vi "TEST_ALL.vi"() -> ()   [LabVIEW 2013]
uses:
  Test State.ctl
  ValveDefaults.ctl
  <vilib>/DAQmx/read.llb/DAQmx Read (Counter DBL 1Chan 1Samp).vi
  <vilib>/DAQmx/read.llb/DAQmx Read (Analog 1D Wfm NChan NSamp).vi
  <vilib>/DAQmx/configure/timing.llb/DAQmx Timing (Sample Clock).vi
  <vilib>/DAQmx/miscellaneous.llb/DAQmx Fill In Error Info.vi
panel:
  in  "Fuel Type":enum16{"RP1", "Biodiesel", "Water"}(ring)=enum."Biodiesel"
  in  "Oxidizer Type":enum16{"LOX", "Water", "Nitrogen"}(ring)
  out "Specific Impulse Display":waveform(dbl)(graph)={"t0"=timestamp(3577994788.047329 s since 1904-01-01), "dt"=0.001, "Y"=[0.0, 0.0, 0.0, 0.0, 0.0, 0.0, 0.0, 0.0, 0.0, 0.0, 0.0, 0.0, 0.0, 0.0, 0.0, 0.0, 0.0, 0.0, 0.0, 0.0, 0.0, 0.0, 0.0, 0.0, 0.0, 0.0, 0.0, 0.0, 0.0, 0.0, 0.0, 0.0, 0.0, 0.0, 0.0, 0.0, 0.0, 0.0, 0.0, 0.0, 0.0, 0.0, 0.0, 0.0, 0.0, 0.0, 0.0, 0.0, 0.0, 0.0, 0.0, 0.0, 0.0, 0.0, 0.0, 0.0, 0.0, 0.0, 0.0, 0.0, 0.0, 0.0, 0.0, 0.0, 0.0, 0.0, 0.0, 0.0, 0.0, 0.0, 0.0, 0.0, 0.0, 0.0, 0.0, 0.0, 0.0, 0.0, 0.0, 0.0, 0.0, 0.0, 0.0, 0.0, 0.0, 0.0, 0.0, 0.0, 0.0, 0.0, 0.0, 0.0, 0.0, 0.0, 0.0, 0.0, 0.0, 0.0, 0.0, 0.0], "attributes"=variant("NI_ChannelName"=variant(string "Loadcell5k"), "NI_UnitDescription"=variant(string "lbs"))} caption="Measurement"
  in  "Burn Time":dbl=6.0
  out "LOX Rate":dbl
  out "Fuel Rate":dbl
  in  "Loop Freq (Hz)":i32=10
  out "LOX Flow Count":dbl
  out "Fuel Flow Count":dbl
  in  "Maximum Pressures":dbl[](array[numeric])=[600.0, 600.0, 600.0, 600.0, 600.0]
  out "Engine Pressure":waveform(dbl)(graph)={"t0"=timestamp(3577994788.047329 s since 1904-01-01), "dt"=0.001, "Y"=[0.0, 0.0, 0.0, 0.0, 0.0, 0.0, 0.0, 0.0, 0.0, 0.0, 0.0, 0.0, 0.0, 0.0, 0.0, 0.0, 0.0, 0.0, 0.0, 0.0, 0.0, 0.0, 0.0, 0.0, 0.0, 0.0, 0.0, 0.0, 0.0, 0.0, 0.0, 0.0, 0.0, 0.0, 0.0, 0.0, 0.0, 0.0, 0.0, 0.0, 0.0, 0.0, 0.0, 0.0, 0.0, 0.0, 0.0, 0.0, 0.0, 0.0, 0.0, 0.0, 0.0, 0.0, 0.0, 0.0, 0.0, 0.0, 0.0, 0.0, 0.0, 0.0, 0.0, 0.0, 0.0, 0.0, 0.0, 0.0, 0.0, 0.0, 0.0, 0.0, 0.0, 0.0, 0.0, 0.0, 0.0, 0.0, 0.0, 0.0, 0.0, 0.0, 0.0, 0.0, 0.0, 0.0, 0.0, 0.0, 0.0, 0.0, 0.0, 0.0, 0.0, 0.0, 0.0, 0.0, 0.0, 0.0, 0.0, 0.0], "attributes"=variant("NI_ChannelName"=variant(string "Loadcell5k"), "NI_UnitDescription"=variant(string "lbs"))} caption="Measurement"
  in  "Write Data Button":bool
  out "Test Message":string
  in  "Start Test Button":bool
  in  "Abort Button":bool
  out "Armed Light":bool
  in  "Fire Button":bool
  in  "ARM TEST":bool
  out "Test State":T1
  out "Load Cell Display":waveform(dbl)(graph) caption="Measurement"
  out "Thermocouple 2 Num":dbl
  out "Thermocouple 1 Num":dbl
  in  "Max Temp 2":dbl=500.0
  in  "Max Temp 1":dbl=500.0
  out "LOX Temp":dbl(slide) scale=-200.0..-100.0
  out "Fuel Temp":dbl(slide) scale=-50.0..50.0
  out "Caution 3":bool
  out "Overtemp Alert":bool
  out "Caution 2":bool
  out "Saving Data Alert":bool
  out "Overpressure Alert":bool
  in  "Analog Data Filepath":path=path "C:/MAE155B-Data/analog-test-data.lvm"
  in  "Sample Rate":dbl=1000.0 caption="Analog Rate (Hz)" format="%0.2f"
  in  "Samples to Read":i32=100 caption="Analog Samples"
  out "LOX Dome Pressure":dbl(knob) scale=0.0..600.0
  out "Fuel Dome Pressure":dbl(knob) scale=0.0..600.0
  out "LOX Tank Pressure":dbl(knob) scale=0.0..600.0
  out "Fuel Tank Pressure":dbl(knob) scale=0.0..600.0
  out "AIR BLEED STATUS":bool
  in  "STOP ALL BUTTON 2":bool
  out "LOX VALVE STATUS":bool
  out "LOX DOME OUT STATUS":bool
  out "LOX DOME IN STATUS":bool
  out "VENT STATUS":bool
  out "FUEL VALVE STATUS":bool
  out "FUEL DOME OUT STATUS":bool
  out "FUEL DOME IN STATUS":bool
  in  "LOX DOME IN":bool
  in  "LOX DOME OUT":bool
  in  "AIR BLEED":bool=TRUE
  in  "FUEL DOME IN":bool
  in  "VENT":bool=TRUE
  in  "LOX VALVE":bool
  in  "FUEL DOME OUT":bool
  in  "FUEL VALVE":bool
  out "LOX Tank (gal)":dbl(slide) scale=0.0..3.0
  out "Fuel Tank (gal)":dbl(slide) scale=0.0..3.0
  # "VALVES WILL DEFAULT TO THEIR \"IDLE\" (NOT FAILURE) STATES WHEN PROGRAM STARTS.\nPRESS \"STOP ALL\" OR \"ABORT\" TO SEND VALVES TO THEIR FAILURE (NOT NECESSARILY UNPOWERED) STATES."
  # "DATA CONFIG"
  # "ANNUNCIATOR"
  # "All lights must be OFF before starting test!"
  # "TANK LEVELS"
  # "TEMPERATURES"
  # "VALVE CONTROL"
  # "TANK PRESSURE"
  # "EN"
  # "FT"
  # "FD"
  # "LT"
  # "LD"
  # "ENGINE PRESSURE"
  # "LOAD CELL"
  # "TEST STATE"
  # "MESSAGE"
  # "SPECIFIC IMPULSE"
  # "ARM TEST"
  # "TO DO: Fix the range on Isp graph!"
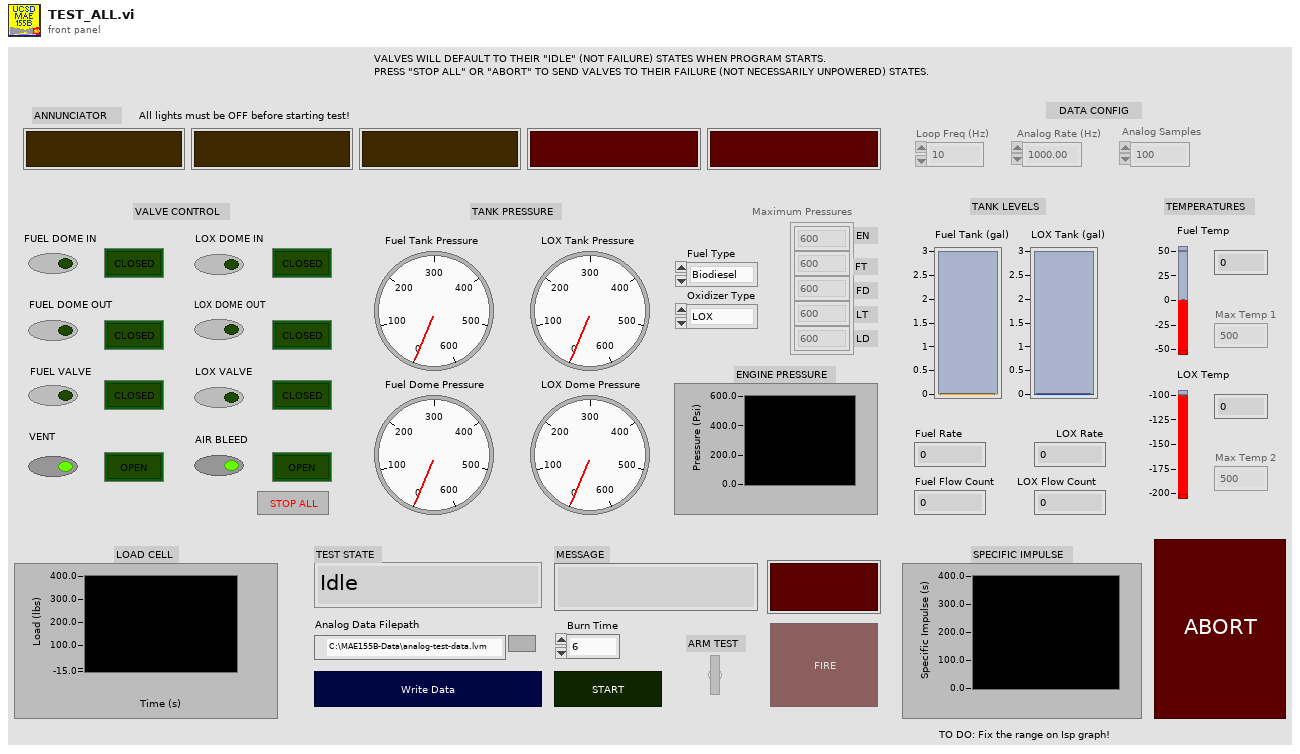
[diagram p1: front panel]
types:
  T1 = typedef "Test State.ctl" = enum16{"Idle", "Start", "LOX Valve Open", "Valve Open Wait", "Fuel Valve Open", "Burn Wait", "LOX Valve Close", "Valve Close Wait", "Fuel Valve Close", "Zero Dome", "Zero Wait", "Vent Valves Open", "Cooldown", "End"}
  T2 = typedef "ValveDefaults.ctl" = bool[]
  T3 = enum8{"Enabled", "Disabled", "Disabled and Grayed Out"}
  T4 = enum16{"NULL", "Caution Data", "Caution 2", "Caution 3", "Warning OverTemp", "Warning OverPressure"}
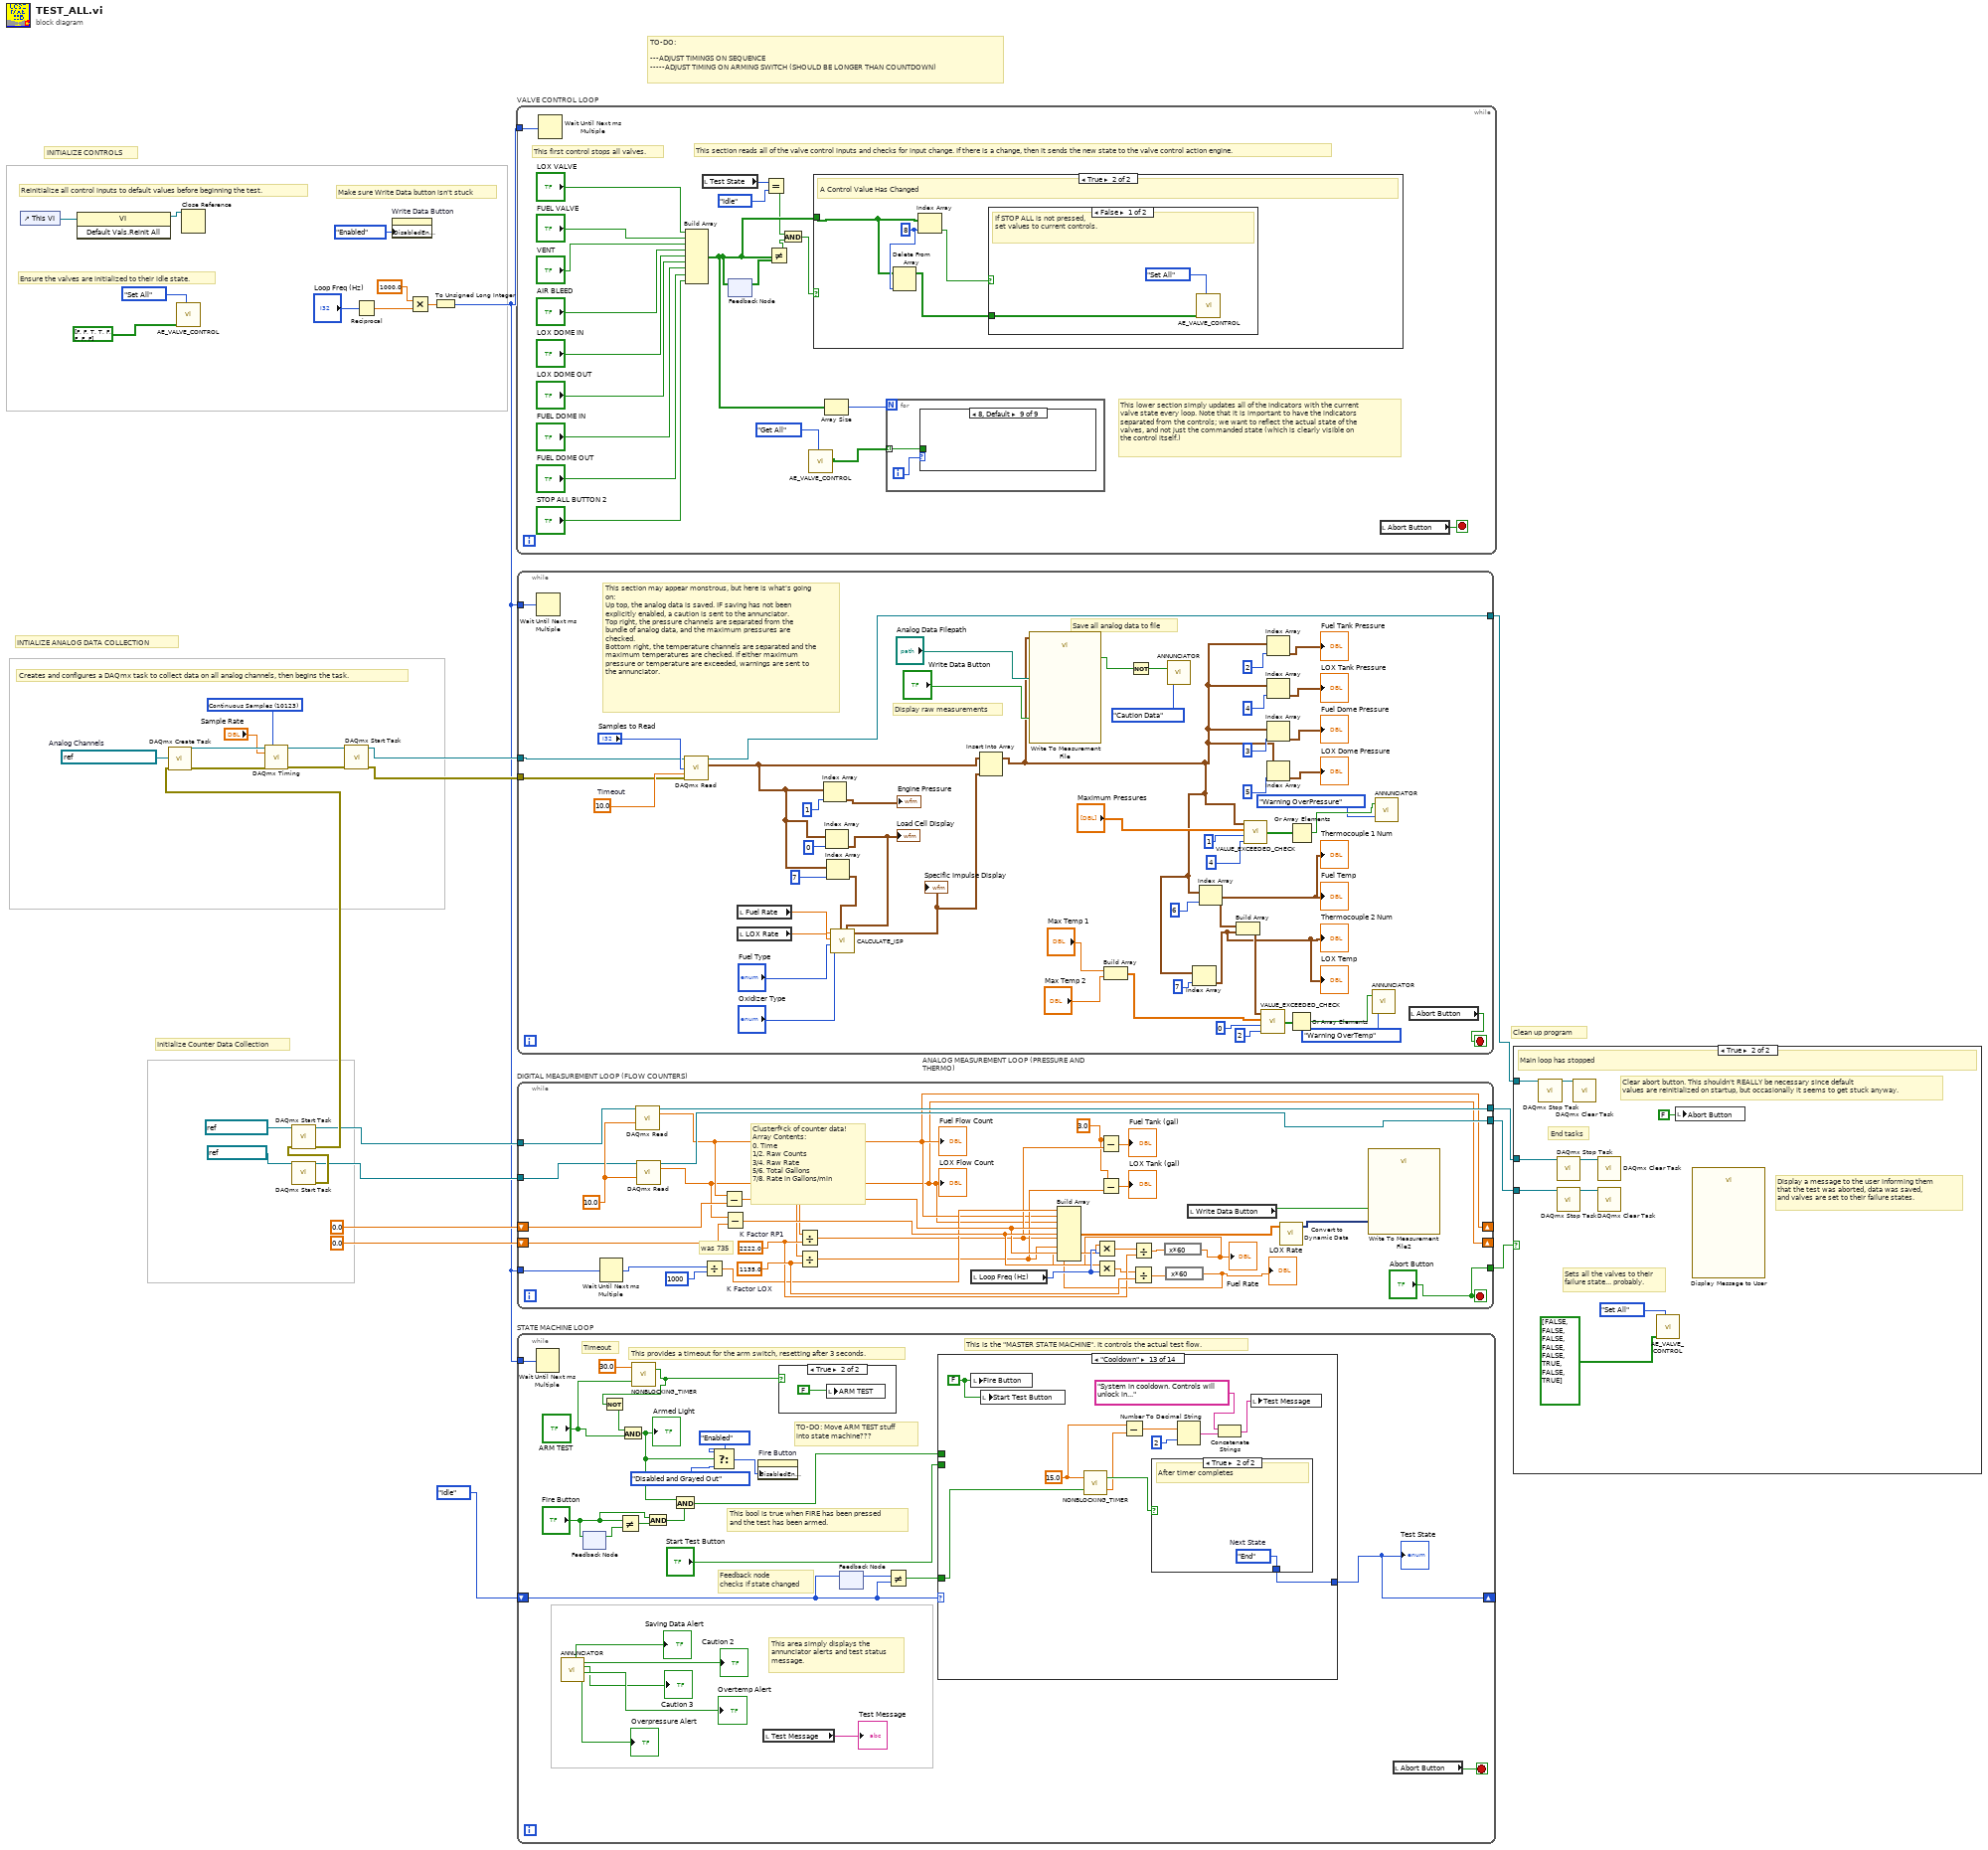
[diagram p0: block diagram]
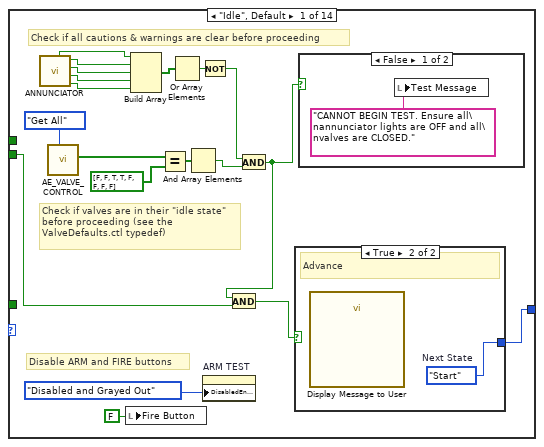
[diagram p2: hidden frame]
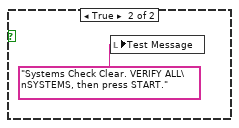
[diagram p3: hidden frame]
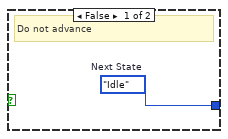
[diagram p4: hidden frame]
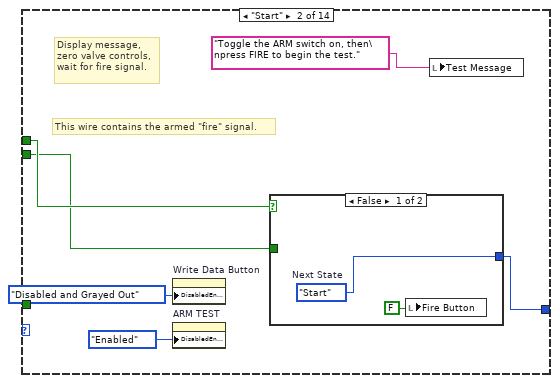
[diagram p5: hidden frame]
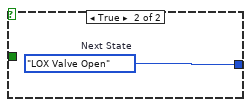
[diagram p6: hidden frame]
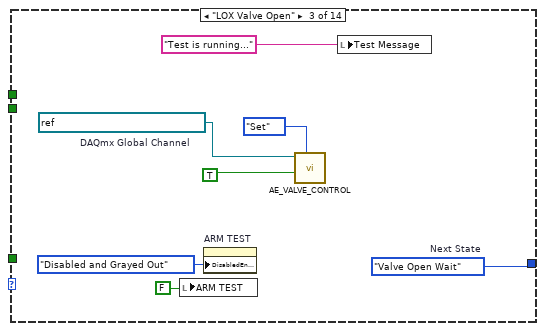
[diagram p7: hidden frame]
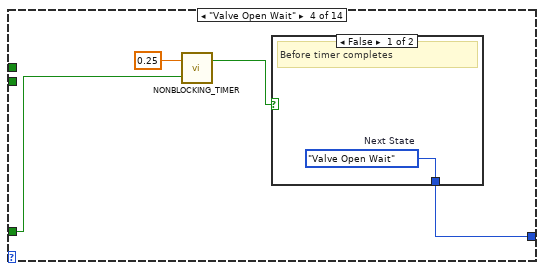
[diagram p8: hidden frame]
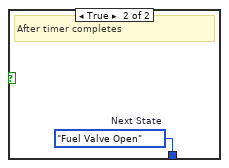
[diagram p9: hidden frame]
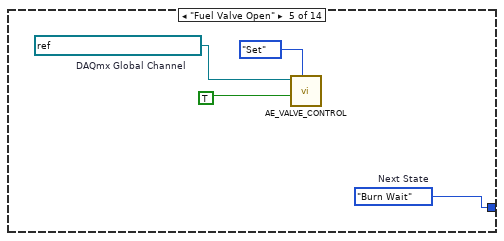
[diagram p10: hidden frame]
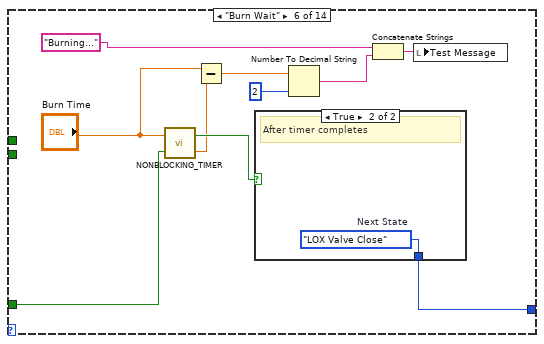
[diagram p11: hidden frame]
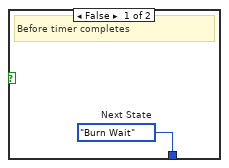
[diagram p12: hidden frame]
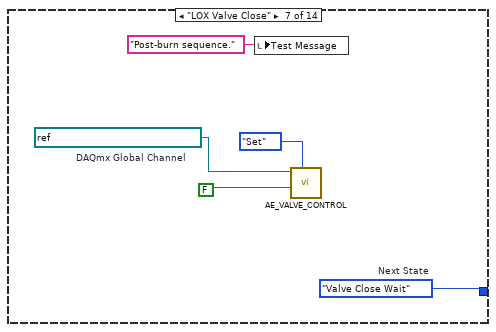
[diagram p13: hidden frame]
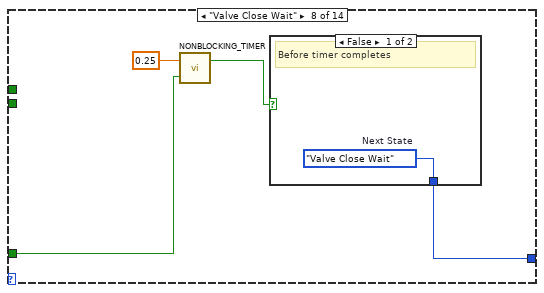
[diagram p14: hidden frame]
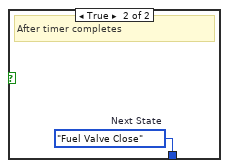
[diagram p15: hidden frame]
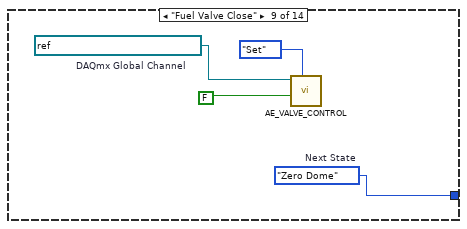
[diagram p16: hidden frame]
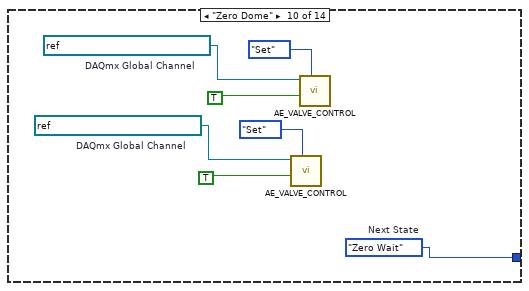
[diagram p17: hidden frame]
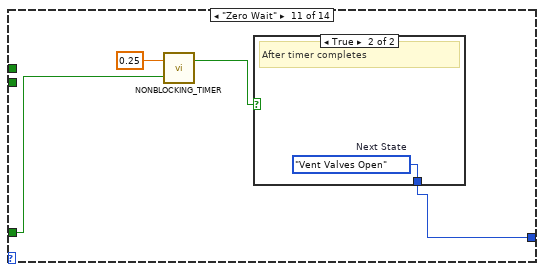
[diagram p18: hidden frame]
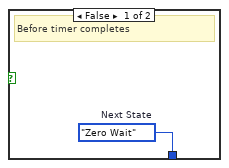
[diagram p19: hidden frame]
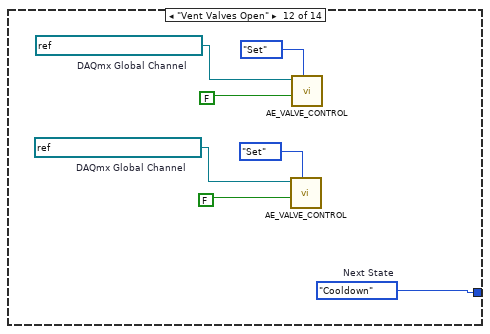
[diagram p20: hidden frame]
diagram:
  w14 = refnum<k21> "Loadcell5k, PRESSURE_ENGINE, PRESSURE_FUEL, PRESSURE_FUEL_DOME, PRESSURE_LOX, PRESSURE_LOX_DOME, THERMO_FUEL, THERMO_LOX"  # Analog Channels
  w30 = 10123 items=["Finite Samples"=10178, "Continuous Samples"=10123] ("sample mode")
  # "Make sure Write Data button isn't stuck"
  # "Ensure the valves are initialized to their idle state."
  # "Initialize Counter Data Collection"
  # "TO-DO:\n\n---ADJUST TIMINGS ON SEQUENCE\n-----ADJUST TIMING ON ARMING SWITCH (SHOULD BE LONGER THAN COUNTDOWN)"
  # "INITIALIZE CONTROLS"
  # "Clean up program"
  # "Reinitialize all control inputs to default values before beginning the test."
  # "Creates and configures a DAQmx task to collect data on all analog channels, then begins the task."
  # "INTIALIZE ANALOG DATA COLLECTION"
  n1 = control-ref of="This VI"() -> (w26:refnum<vi>)
  n2 = invoke class="VI" method="Default Vals.Reinit All"(reference=w26) -> (reference out=w25:refnum<vi>)  [unwired: 2 in, 2 out]
  n3 = call "AE_VALVE_CONTROL.vi"("Action"=enum16{"Set", "Set All", "Get", "Get All"}."Set All", "Array In"=T2 [FALSE, FALSE, TRUE, TRUE, FALSE, FALSE, FALSE, FALSE] ("Array")) -> ()  [unwired: 8 in, 2 out]
  n4 = Close Reference(reference=w25) -> ()  [unwired: 1 in, 1 out]
  n5 = call <vilib>:"DAQmx Start Task.vi"("task/channels in"=refnum<k21> "TFM_LOX" ("Global Virtual Channels AI 2")) -> ("task out"=w10:refnum<k21>, "error out"=w15:errorcluster)  [unwired: 13 in]
  n6 = call <vilib>:"DAQmx Start Task.vi"("task/channels in"=refnum<k21> "TFM_FUEL" ("Global Virtual Channels AI 2"), "error in"=w15) -> ("task out"=w11:refnum<k21>, "error out"=w23:errorcluster)  [unwired: 12 in]
  n7 = call <vilib>:"DAQmx Create Task.vi"("global virtual channels"=w14, "error in"=w23) -> ("task out"=w31:refnum<k21>, "error out"=w32:errorcluster)  [unwired: 12 in]
  n8 = call-poly <vilib>:"DAQmx Timing.vi"("task/channels in"=w31, "sample mode"=w30, "rate"="Sample Rate", "error in"=w32) -> ("task out"=w29:refnum<k21>, "error out"=w28:errorcluster)  [unwired: 10 in]
  n9 = call <vilib>:"DAQmx Start Task.vi"("task/channels in"=w29, "error in"=w28) -> ("task out"=w13:refnum<k21>, "error out"=w12:errorcluster)  [unwired: 12 in]
  n10 = Reciprocal(x="Loop Freq (Hz)") -> (1/x=w19:dbl)
  n11 = property on="Write Data Button" class="Bool (strict)"("DisabledEnum"=T3."Enabled" ("Disabled")) -> ()  [unwired: 2 in, 2 out]
  n12 = Multiply(x=1000.0, y=w19) -> (x*y=w18:dbl)
  n13 = To Unsigned Long Integer(number=w18) -> (unsigned 32bit integer=w2:u32)
  n14 = while "VALVE CONTROL LOOP" {
    tunnel: w2 -> [w33]
    stop <- w34 stop-if-true
    # "This lower section simply updates all of the indicators with the current\nvalve state every loop. Note that it is important to have the indicators\nseparated from the controls; we want to reflect the actual state of the\nvalves, and not just the commanded state (which is clearly visible on \nthe control itself.)"
    # "This first control stops all valves."
    # "This section reads all of the valve control inputs and checks for input change. If there is a change, then it sends the new state to the valve control action engine."
    n15 = Wait Until Next ms Multiple(millisecond multiple=w33) -> ()  [unwired: 1 out]
    n16 = Build Array("LOX VALVE", "FUEL VALVE", "VENT", "AIR BLEED", "LOX DOME IN", "LOX DOME OUT", "FUEL DOME IN", "FUEL DOME OUT", "STOP ALL BUTTON 2") -> (w51:bool[])
    n17 = local read "Test State"() -> (w45:T1)
    n18 = feedback-in #1(w51) -> ()
    n19 = feedback #1() -> (w53:bool[])  [unwired: 1 in]
    n20 = Equal?(x=w45, y=Test_State."Idle" ("Test State")) -> (x = y?=w44:bool)
    n21 = Not Equal?(x=w51, y=w53) -> (x != y?=w47:bool)
    n22 = And(x=w44, y=w47) -> (x .and. y?=w48:bool)
    n23 = call "AE_VALVE_CONTROL.vi"("Action"=enum16{"Set", "Set All", "Get", "Get All"}."Get All") -> ("All Channel Status"=w49:bool[])  [unwired: 9 in, 1 out]
    n24 = case shown="True" w48 {
      tunnel: w51 -> [_ w65]
      frame False {
        # "Controls Have Not Changed"
      }
      frame True {
        w66 = 8
        # "A Control Value Has Changed"
        n25 = Delete From Array(array=w65, index=w66) -> (array with subset deleted=w64:bool[])  [unwired: 1 in, 1 out]
        n26 = Index Array(array=w65, index=w66) -> (element=w67:bool)
        n27 = case shown="False" w67 {
          tunnel: w64 -> [w68 _]
          frame False {
            # "If STOP ALL is not pressed,\nset values to current controls."
            n28 = call "AE_VALVE_CONTROL.vi"("Action"=enum16{"Set", "Set All", "Get", "Get All"}."Set All", "Array In"=w68) -> ()  [unwired: 8 in, 2 out]
          }
          frame True {
            # "If STOP ALL is pressed,\nset all valves to FALSE."
            n29 = call "AE_VALVE_CONTROL.vi"("Action"=enum16{"Set", "Set All", "Get", "Get All"}."Set All", "Array In"=T2 [FALSE, FALSE, FALSE, FALSE, FALSE, FALSE, FALSE, FALSE]) -> ()  [unwired: 8 in, 2 out]
          }
        }
      }
    }
    n30 = Array Size(array=w51) -> (size(s)=w52:i32)
    n31 = for {
      N: w52 -> [_]
      tunnel: w49 -> [w54] mode=indexing
      i -> [w55]
      n32 = case shown="8, Default" w55 {
        tunnel: w54 -> [w56 w57 w58 w59 w60 w61 w62 w63 _]
        frame 0 {
          "LOX VALVE STATUS" <- w56
        }
        frame 1 {
          "FUEL VALVE STATUS" <- w57
        }
        frame 2 {
          "VENT STATUS" <- w58
        }
        frame 3 {
          "AIR BLEED STATUS" <- w59
        }
        frame 4 {
          "LOX DOME IN STATUS" <- w60
        }
        frame 5 {
          "LOX DOME OUT STATUS" <- w61
        }
        frame 6 {
          "FUEL DOME IN STATUS" <- w62
        }
        frame 7 {
          "FUEL DOME OUT STATUS" <- w63
        }
        frame 8, Default {
        }
      }
    }
    n33 = local read "Abort Button"() -> (w34:bool)
  }
  n34 = while "ANALOG MEASUREMENT LOOP (PRESSURE AND THERMO)" {
    tunnel: w13 -> [w91]
    tunnel: w12 -> [w90]
    tunnel: [w89] -> w7
    tunnel: w2 -> [w87]
    stop <- w88 stop-if-true
    w100 = 10.0  # Timeout
    # "This section may appear monstrous, but here is what's going on:\nUp top, the analog data is saved. IF saving has not been explicitly enabled, a caution is sent to the annunciator.\nTop right, the pressure channels are separated from the bundle of analog data, and the maximum pressures are checked.\nBottom right, the temperature channels are separated and the maximum temperatures are checked. If either maximum pressure or temperature are exceeded, warnings are sent to the annunciator."
    # "Save all analog data to file"
    # "Display raw measurements"
    n35 = Wait Until Next ms Multiple(millisecond multiple=w87) -> ()  [unwired: 1 out]
    n36 = call-poly <vilib>:"DAQmx Read.vi"("task/channels in"=w91, "number of samples per channel"="Samples to Read", "timeout"=w100, "error in"=w90) -> ("task out"=w89:refnum<k21>, "data"=w75:waveform(dbl)[])  [unwired: 9 in, 1 out]
    n37 = local read "Fuel Rate"() -> (w84:dbl)
    n38 = local read "LOX Rate"() -> (w85:dbl)
    n39 = Index Array(array=w75, index=1) -> (element=→"Engine Pressure":waveform(dbl))
    n40 = Index Array(array=w75, index=0) -> (element=w72:waveform(dbl))
    "Load Cell Display" <- w72
    n41 = Index Array(array=w75, index=7) -> (element=w80:waveform(dbl))
    n42 = call "CALCULATE_ISP.vi"("Thrust"=w72, "Oxidizer Temperature"=w80, "Oxidizer Type"="Oxidizer Type", "Fuel Type"="Fuel Type", "Oxidizer Flow Rate"=w85, "Fuel Flow Rate"=w84) -> ("Specific Impulse"=w74:waveform(dbl))  [unwired: 5 in]
    "Specific Impulse Display" <- w74
    n43 = Insert Into Array(array=w75, new element=w74) -> (w76:waveform(dbl)[])  [unwired: 1 in]
    n44 = call "Write To Measurement File"("Signals"=w76, "Enable"="Write Data Button", "Filename"="Analog Data Filepath") -> ("Saving Data"=w103:bool)  [unwired: 14 in, 2 out]
    n45 = Build Array("Max Temp 1", "Max Temp 2") -> (w82:dbl[])
    n46 = Not(x=w103) -> (.not. x?=w117:bool)
    n47 = call "ANNUNCIATOR.vi"("Input Channel"=T4."Caution Data", "Input Value"=w117) -> ()  [unwired: 5 out]
    n48 = Index Array(array=w76, index=7) -> (element=w83:waveform(dbl))
    "LOX Temp" <- w83
    "Thermocouple 2 Num" <- w83
    n49 = Index Array(array=w76, index=6) -> (element=w112:waveform(dbl))
    "Fuel Temp" <- w112
    "Thermocouple 1 Num" <- w112
    n50 = Build Array(w112, w83) -> (w113:waveform(dbl)[])
    n51 = call "VALUE_EXCEEDED_CHECK.vi"("Number of Channels"=4, "Start Channel Index"=1, "Max Value Array"="Maximum Pressures", "Input Array"=w76) -> ("Array"=w106:bool[])
    n52 = call "VALUE_EXCEEDED_CHECK.vi"("Number of Channels"=2, "Start Channel Index"=0, "Max Value Array"=w82, "Input Array"=w113) -> ("Array"=w109:bool[])
    n53 = Index Array(array=w76, index=2) -> (element=→"Fuel Tank Pressure":waveform(dbl))
    n54 = Index Array(array=w76, index=4) -> (element=→"LOX Tank Pressure":waveform(dbl))
    n55 = Index Array(array=w76, index=3) -> (element=→"Fuel Dome Pressure":waveform(dbl))
    n56 = Index Array(array=w76, index=5) -> (element=→"LOX Dome Pressure":waveform(dbl))
    n57 = Or Array Elements(Boolean array=w109) -> (logical OR=w116:bool)
    n58 = Or Array Elements(Boolean array=w106) -> (logical OR=w121:bool)
    n59 = call "ANNUNCIATOR.vi"("Input Channel"=T4."Warning OverTemp", "Input Value"=w116) -> ()  [unwired: 5 out]
    n60 = call "ANNUNCIATOR.vi"("Input Channel"=T4."Warning OverPressure", "Input Value"=w121) -> ()  [unwired: 5 out]
    n61 = local read "Abort Button"() -> (w88:bool)
  }
  n62 = while "DIGITAL MEASUREMENT LOOP (FLOW COUNTERS)" {
    tunnel: w11 -> [w136]
    tunnel: w10 -> [w135]
    tunnel: w2 -> [w134]
    tunnel: [w131] -> w6
    tunnel: [w130] -> w5
    shift-right: [w129] -> _
    shift-left: 0.0 -> [w133]
    shift-right: [w128] -> _
    shift-left: 0.0 -> [w132]
    tunnel: ["Abort Button"] -> w3
    stop <- "Abort Button" stop-if-true
    w154 = 1135.0  # K Factor LOX
    w144 = 3.0
    w153 = 2222.0  # K Factor RP1
    w138 = 10.0 ("timeout")
    # "was 735"
    # "Clusterf*ck of counter data!\nArray Contents:\n0. Time\n1/2. Raw Counts\n3/4. Raw Rate\n5/6. Total Gallons\n7/8. Rate in Gallons/min"
    n63 = Wait Until Next ms Multiple(millisecond multiple=w134) -> (millisecond timer value=w141:u32)
    n64 = call-poly <vilib>:"DAQmx Read.vi"("task/channels in"=w136, "timeout"=w138) -> ("task out"=w131:refnum<k21>, "data"=w129:dbl)  [unwired: 11 in, 1 out]
    "Fuel Flow Count" <- w129
    n65 = call-poly <vilib>:"DAQmx Read.vi"("task/channels in"=w135, "timeout"=w138) -> ("task out"=w130:refnum<k21>, "data"=w128:dbl)  [unwired: 11 in, 1 out]
    "LOX Flow Count" <- w128
    n66 = Divide(x=w141, y=1000) -> (x/y=w147:dbl)
    n67 = Subtract(x=w129, y=w133) -> (x-y=w148:dbl)
    n68 = Subtract(x=w128, y=w132) -> (x-y=w149:dbl)
    n69 = Divide(x=w129, y=w153) -> (x/y=w145:dbl)
    n70 = Divide(x=w128, y=w154) -> (x/y=w146:dbl)
    n71 = local read "Loop Freq (Hz)"() -> (w150:i32)
    n72 = Multiply(x=w148, y=w150) -> (x*y=w151:dbl)
    n73 = Multiply(x=w149, y=w150) -> (x*y=w152:dbl)
    n74 = Subtract(x=w144, y=w145) -> (x-y=→"Fuel Tank (gal)":dbl)
    n75 = Subtract(x=w144, y=w146) -> (x-y=→"LOX Tank (gal)":dbl)
    n76 = Divide(x=w152, y=w154) -> (x/y=w156:dbl)
    n77 = Divide(x=w151, y=w153) -> (x/y=w155:dbl)
    n78 = expression code="x*60"(w155) -> (w124:dbl)
    "Fuel Rate" <- w124
    n79 = expression code="x*60"(w156) -> (w125:dbl)
    "LOX Rate" <- w125
    n80 = Build Array(w147, w129, w128, w148, w149, w145, w146, w124, w125) -> (w139:dbl[])
    n81 = local read "Write Data Button"() -> (w137:bool)
    n82 = call "Convert to Dynamic Data"("Array"=w139) -> ("Dynamic Data Type"=w126:dynamicdata)  [unwired: 3 in]
    n83 = call "Write To Measurement File2"("Signals"=w126, "Enable"=w137) -> ()  [unwired: 15 in, 3 out]
  }
  n84 = while "STATE MACHINE LOOP" {
    shift-right: [w160] -> _
    shift-left: Test_State."Idle" ("Test State") -> [w162]
    tunnel: w2 -> [w157]
    stop <- w161 stop-if-true
    # "Timeout"
    # "This is the \"MASTER STATE MACHINE\". It controls the actual test flow."
    # "TO-DO: Move ARM TEST stuff\ninto state machine???"
    # "This area simply displays the\nannunciator alerts and test status\nmessage."
    # "Feedback node\nchecks if state changed"
    # "This bool is true when FIRE has been pressed\nand the test has been armed."
    # "This provides a timeout for the arm switch, resetting after 3 seconds."
    n85 = Wait Until Next ms Multiple(millisecond multiple=w157) -> ()  [unwired: 1 out]
    n86 = call "ANNUNCIATOR.vi"() -> ("Out Warning OverPressure"=→"Overpressure Alert":bool, "Out Warning OverTemp"=→"Overtemp Alert":bool, "Out Caution 3"=→"Caution 3":bool, "Out Caution 2"=→"Caution 2":bool, "Out Caution Data"=→"Saving Data Alert":bool)  [unwired: 2 in]
    n87 = feedback #2() -> (w165:bool)  [unwired: 1 in]
    n88 = feedback-in #2("Fire Button") -> ()
    n89 = Not Equal?(x="Fire Button", y=w165) -> (x != y?=w166:bool)
    n90 = call "NONBLOCKING_TIMER.vi"("Start on Value Changed"="ARM TEST", "Time to Wait"=30.0) -> ("Timer Has Elapsed"=w159:bool)  [unwired: 1 out]
    n91 = Not(x=w159) -> (.not. x?=w164:bool)
    n92 = And(x=w164, y="ARM TEST") -> (x .and. y?=w179:bool)
    "Armed Light" <- w179
    n93 = And(x="Fire Button", y=w166) -> (x .and. y?=w168:bool)
    n94 = And(x=w179, y=w168) -> (x .and. y?=w169:bool)
    n95 = Select(t=T3."Enabled" ("Disabled"), s=w179, f=T3."Disabled and Grayed Out" ("Disabled")) -> (s? t:f=w182:T3)
    n96 = property on="Fire Button" class="Bool (strict)"("DisabledEnum"=w182) -> ()  [unwired: 2 in, 2 out]
    n97 = local read "Test Message"() -> (→"Test Message":string)
    n98 = case shown="True" w159 {
      frame False {
      }
      frame True {
        n99 = local write "ARM TEST"(FALSE) -> ()
      }
    }
    n100 = feedback #3() -> (w177:T1)  [unwired: 1 in]
    n101 = feedback-in #3(w162) -> ()
    n102 = Not Equal?(x=w177, y=w162) -> (x != y?=w178:bool)
    n103 = case shown="\"Cooldown\"" w162 {
      tunnel: [w201 w210 w220 w225 w231 w240 w245 w250 w255 w265 w267 w272 w287 w297] -> w160
      tunnel: w169 -> [_ w211 _ _ _ _ _ _ _ _ _ _ _ _]
      tunnel: "Start Test Button" -> [w186 w206 _ _ _ _ _ _ _ _ _ _ _ _]
      tunnel: w178 -> [_ _ _ w222 _ w239 _ w249 _ _ w266 _ w286 _]
      frame "Idle", Default {
        # "Check if valves are in their \"idle state\"\nbefore proceeding (see the\nValveDefaults.ctl typedef)"
        # "Check if all cautions & warnings are clear before proceeding"
        # "Disable ARM and FIRE buttons"
        n104 = call "ANNUNCIATOR.vi"() -> ("Out Warning OverPressure"=w194:bool, "Out Warning OverTemp"=w195:bool, "Out Caution 3"=w196:bool, "Out Caution 2"=w197:bool, "Out Caution Data"=w198:bool)  [unwired: 2 in]
        n105 = call "AE_VALVE_CONTROL.vi"("Action"=enum16{"Set", "Set All", "Get", "Get All"}."Get All") -> ("All Channel Status"=w184:bool[])  [unwired: 9 in, 1 out]
        n106 = local write "Fire Button"(FALSE) -> ()
        n107 = Build Array(w198, w197, w196, w195, w194) -> (w200:bool[])
        n108 = Equal?(x=w184, y=T2 [FALSE, FALSE, TRUE, TRUE, FALSE, FALSE, FALSE, FALSE] ("Array")) -> (x = y?=w189:T2)
        n109 = Or Array Elements(Boolean array=w200) -> (logical OR=w199:bool)
        n110 = And Array Elements(Boolean array=w189) -> (logical AND=w190:bool)
        n111 = Not(x=w199) -> (.not. x?=w188:bool)
        n112 = property on="ARM TEST" class="Bool (strict)"("DisabledEnum"=T3."Disabled and Grayed Out" ("Disabled")) -> ()  [unwired: 2 in, 2 out]
        n113 = And(x=w188, y=w190) -> (x .and. y?=w187:bool)
        n114 = And(x=w187, y=w186) -> (x .and. y?=w185:bool)
        n115 = case shown="True" w185 {
          tunnel: [w204 w205] -> w201
          frame False {
            w204 = Test_State."Idle"  # Next State
            # "Do not advance"
          }
          frame True {
            w205 = Test_State."Start"  # Next State
            # "Advance"
            n116 = call "Display Message to User"() -> ()  [unwired: 10 in, 2 out]
          }
        }
        n117 = case shown="False" w187 {
          frame False {
            n118 = local write "Test Message"("CANNOT BEGIN TEST. Ensure all\nannunciator lights are OFF and all\nvalves are CLOSED.") -> ()
          }
          frame True {
            n119 = local write "Test Message"("Systems Check Clear. VERIFY ALL\nSYSTEMS, then press START.") -> ()
          }
        }
      }
      frame "Start" {
        # "Display message,\nzero valve controls,\nwait for fire signal."
        # "This wire contains the armed \"fire\" signal."
        n120 = property on="Write Data Button" class="Bool (strict)"("DisabledEnum"=T3."Disabled and Grayed Out" ("Disabled")) -> ()  [unwired: 2 in, 2 out]
        n121 = property on="ARM TEST" class="Bool (strict)"("DisabledEnum"=T3."Enabled" ("Disabled")) -> ()  [unwired: 2 in, 2 out]
        n122 = case shown="False" w211 {
          tunnel: [w212 w214] -> w210
          tunnel: w206 -> [_ _]
          frame False {
            w212 = Test_State."Start"  # Next State
            n123 = local write "Fire Button"(FALSE) -> ()
          }
          frame True {
            w214 = Test_State."LOX Valve Open"  # Next State
          }
        }
        n124 = local write "Test Message"("Toggle the ARM switch on, then\npress FIRE to begin the test.") -> ()
      }
      frame "LOX Valve Open" {
        w218 = refnum<k21> "LOX_VALVE"  # DAQmx Global Channel
        w220 = Test_State."Valve Open Wait"  # Next State
        n125 = local write "ARM TEST"(FALSE) -> ()
        n126 = property on="ARM TEST" class="Bool (strict)"("DisabledEnum"=T3."Disabled and Grayed Out" ("Disabled")) -> ()  [unwired: 2 in, 2 out]
        n127 = call "AE_VALVE_CONTROL.vi"("Action"=enum16{"Set", "Set All", "Get", "Get All"}."Set", "Bool In"=TRUE, "DAQmx Global Channel"=w218) -> ()  [unwired: 7 in, 2 out]
        n128 = local write "Test Message"("Test is running...") -> ()
      }
      frame "Valve Open Wait" {
        n129 = call "NONBLOCKING_TIMER.vi"("Start on Value Changed"=w222, "Time to Wait"=0.25) -> ("Timer Has Elapsed"=w224:bool)  [unwired: 1 out]
        n130 = case shown="False" w224 {
          tunnel: [w226 w227] -> w225
          frame False {
            w226 = Test_State."Valve Open Wait"  # Next State
            # "Before timer completes"
          }
          frame True {
            w227 = Test_State."Fuel Valve Open"  # Next State
            # "After timer completes"
          }
        }
      }
      frame "Fuel Valve Open" {
        w229 = refnum<k21> "FUEL_VALVE"  # DAQmx Global Channel
        w231 = Test_State."Burn Wait"  # Next State
        n131 = call "AE_VALVE_CONTROL.vi"("Action"=enum16{"Set", "Set All", "Get", "Get All"}."Set", "Bool In"=TRUE, "DAQmx Global Channel"=w229) -> ()  [unwired: 7 in, 2 out]
      }
      frame "Burn Wait" {
        n132 = call "NONBLOCKING_TIMER.vi"("Start on Value Changed"=w239, "Time to Wait"="Burn Time") -> ("Elapsed Time"=w234:dbl, "Timer Has Elapsed"=w241:bool)
        n133 = Subtract(x="Burn Time", y=w234) -> (x-y=w233:dbl)
        n134 = case shown="True" w241 {
          tunnel: [w242 w243] -> w240
          frame False {
            w242 = Test_State."Burn Wait"  # Next State
            # "Before timer completes"
          }
          frame True {
            w243 = Test_State."LOX Valve Close"  # Next State
            # "After timer completes"
          }
        }
        n135 = Number To Decimal String(number=w233, width (-)=2) -> (decimal integer string=w236:string)
        n136 = Concatenate Strings("Burning...", w236) -> (w238:string)
        n137 = local write "Test Message"(w238) -> ()
      }
      frame "LOX Valve Close" {
        w247 = refnum<k21> "LOX_VALVE"  # DAQmx Global Channel
        w245 = Test_State."Valve Close Wait"  # Next State
        n138 = local write "Test Message"("Post-burn sequence.") -> ()
        n139 = call "AE_VALVE_CONTROL.vi"("Action"=enum16{"Set", "Set All", "Get", "Get All"}."Set", "Bool In"=FALSE, "DAQmx Global Channel"=w247) -> ()  [unwired: 7 in, 2 out]
      }
      frame "Valve Close Wait" {
        n140 = call "NONBLOCKING_TIMER.vi"("Start on Value Changed"=w249, "Time to Wait"=0.25) -> ("Timer Has Elapsed"=w252:bool)  [unwired: 1 out]
        n141 = case shown="False" w252 {
          tunnel: [w253 w254] -> w250
          frame False {
            w253 = Test_State."Valve Close Wait"  # Next State
            # "Before timer completes"
          }
          frame True {
            w254 = Test_State."Fuel Valve Close"  # Next State
            # "After timer completes"
          }
        }
      }
      frame "Fuel Valve Close" {
        w257 = refnum<k21> "FUEL_VALVE"  # DAQmx Global Channel
        w255 = Test_State."Zero Dome"  # Next State
        n142 = call "AE_VALVE_CONTROL.vi"("Action"=enum16{"Set", "Set All", "Get", "Get All"}."Set", "Bool In"=FALSE, "DAQmx Global Channel"=w257) -> ()  [unwired: 7 in, 2 out]
      }
      frame "Zero Dome" {
        w260 = refnum<k21> "LOX_DOME_OUT"  # DAQmx Global Channel
        w263 = refnum<k21> "FUEL_DOME_OUT"  # DAQmx Global Channel
        w265 = Test_State."Zero Wait"  # Next State
        n143 = call "AE_VALVE_CONTROL.vi"("Action"=enum16{"Set", "Set All", "Get", "Get All"}."Set", "Bool In"=TRUE, "DAQmx Global Channel"=w260) -> ()  [unwired: 7 in, 2 out]
        n144 = call "AE_VALVE_CONTROL.vi"("Action"=enum16{"Set", "Set All", "Get", "Get All"}."Set", "Bool In"=TRUE, "DAQmx Global Channel"=w263) -> ()  [unwired: 7 in, 2 out]
      }
      frame "Zero Wait" {
        n145 = call "NONBLOCKING_TIMER.vi"("Start on Value Changed"=w266, "Time to Wait"=0.25) -> ("Timer Has Elapsed"=w269:bool)  [unwired: 1 out]
        n146 = case shown="True" w269 {
          tunnel: [w270 w271] -> w267
          frame False {
            w270 = Test_State."Zero Wait"  # Next State
            # "Before timer completes"
          }
          frame True {
            w271 = Test_State."Vent Valves Open"  # Next State
            # "After timer completes"
          }
        }
      }
      frame "Vent Valves Open" {
        w272 = Test_State."Cooldown"  # Next State
        w274 = refnum<k21> "AIR_BLEED"  # DAQmx Global Channel
        w277 = refnum<k21> "VENT"  # DAQmx Global Channel
        n147 = call "AE_VALVE_CONTROL.vi"("Action"=enum16{"Set", "Set All", "Get", "Get All"}."Set", "Bool In"=FALSE, "DAQmx Global Channel"=w274) -> ()  [unwired: 7 in, 2 out]
        n148 = call "AE_VALVE_CONTROL.vi"("Action"=enum16{"Set", "Set All", "Get", "Get All"}."Set", "Bool In"=FALSE, "DAQmx Global Channel"=w277) -> ()  [unwired: 7 in, 2 out]
      }
      frame "Cooldown" {
        w284 = 15.0
        w289 = FALSE
        n149 = local write "Fire Button"(w289) -> ()
        n150 = local write "Start Test Button"(w289) -> ()
        n151 = call "NONBLOCKING_TIMER.vi"("Start on Value Changed"=w286, "Time to Wait"=w284) -> ("Elapsed Time"=w283:dbl, "Timer Has Elapsed"=w288:bool)
        n152 = Subtract(x=w284, y=w283) -> (x-y=w282:dbl)
        n153 = case shown="True" w288 {
          tunnel: [w290 w291] -> w287
          frame False {
            w290 = Test_State."Cooldown"  # Next State
            # "Before timer completes"
          }
          frame True {
            w291 = Test_State."End"  # Next State
            # "After timer completes"
          }
        }
        n154 = Number To Decimal String(number=w282, width (-)=2) -> (decimal integer string=w281:string)
        n155 = Concatenate Strings("System in cooldown. Controls will unlock in...", w281) -> (w279:string)
        n156 = local write "Test Message"(w279) -> ()
      }
      frame "End" {
        n157 = local read "Start Test Button"() -> (w295:bool)
        n158 = call "AE_VALVE_CONTROL.vi"("Action"=enum16{"Set", "Set All", "Get", "Get All"}."Set All", "Array In"=T2 [FALSE, FALSE, FALSE, FALSE, FALSE, FALSE, FALSE, FALSE]) -> ()  [unwired: 8 in, 2 out]
        n159 = property on="Write Data Button" class="Bool (strict)"("DisabledEnum"=T3."Enabled" ("Disabled")) -> ()  [unwired: 2 in, 2 out]
        n160 = case shown="True" w295 {
          tunnel: [w298 w300] -> w297
          frame False {
            w298 = Test_State."End"  # Next State
          }
          frame True {
            w300 = Test_State."Idle"  # Next State
            n161 = local write "Start Test Button"(FALSE) -> ()
          }
        }
        n162 = local write "Test Message"("Test complete. CONTROLS LOCKED.\nPress START to return to Idle state\nand unlock controls.") -> ()
      }
    }
    "Test State" <- w160
    n163 = local read "Abort Button"() -> (w161:bool)
  }
  n164 = case shown="True" w3 {
    tunnel: w7 -> [_ w309]
    tunnel: w6 -> [_ w305]
    tunnel: w5 -> [_ w303]
    frame False {
      # "Main loop still running"
    }
    frame True {
      # "Display a message to the user informing them\nthat the test was aborted, data was saved,\nand valves are set to their failure states."
      # "Clear abort button. This shouldn't REALLY be necessary since default\nvalues are reinitialized on startup, but occasionally it seems to get stuck anyway."
      # "End tasks"
      # "Sets all the valves to their\nfailure state... probably."
      # "Main loop has stopped"
      n165 = call <vilib>:"DAQmx Stop Task.vi"("task/channels in"=w309) -> ("task out"=w310:refnum<k21>)  [unwired: 13 in, 1 out]
      n166 = call <vilib>:"DAQmx Stop Task.vi"("task/channels in"=w305) -> ("task out"=w304:refnum<k21>)  [unwired: 13 in, 1 out]
      n167 = call <vilib>:"DAQmx Stop Task.vi"("task/channels in"=w303) -> ("task out"=w302:refnum<k21>)  [unwired: 13 in, 1 out]
      n168 = call <vilib>:"DAQmx Clear Task.vi"("task in"=w310) -> ()  [unwired: 14 in, 1 out]
      n169 = call <vilib>:"DAQmx Clear Task.vi"("task in"=w304) -> ()  [unwired: 14 in, 1 out]
      n170 = call <vilib>:"DAQmx Clear Task.vi"("task in"=w302) -> ()  [unwired: 14 in, 1 out]
      n171 = call "AE_VALVE_CONTROL.vi"("Action"=enum16{"Set", "Set All", "Get", "Get All"}."Set All", "Array In"=T2 [FALSE, FALSE, FALSE, FALSE, FALSE, TRUE, FALSE, TRUE]) -> ()  [unwired: 8 in, 2 out]
      n172 = local write "Abort Button"(FALSE) -> ()
      n173 = call "Display Message to User"() -> ()  [unwired: 10 in, 2 out]
    }
  }
